vi "Insert Tag.vi"(0 "Image Data in":u8[](array[numeric]), 2 "Cluster":T1={"Tag"=30, "Type"=enum."RATIONAL", "Count"=2, "Val/Offs"=106, "Is Pointer?"=TRUE, "Byte stream index"=0}, 4 "Litt/BigEnd":bool) -> (5 "Image Data Out":u8[](array[numeric]))   [LabVIEW 2013, in "Tiff reader.lvlib"]
doc: "Sets a tag entry in the Image File Directory in a tiff file byte stream."
uses:
  Tiff reader.lvlib
  IFD Entry.ctl
  FieldTypes.ctl
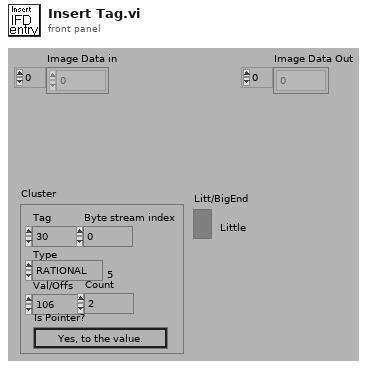
[diagram p1: front panel]
types:
  T1 = typedef "Tiff reader.lvlib/IFD Entry.ctl" = cluster{"Tag":u16, "Type":T2, "Count":u32, "Val/Offs":u32, "Is Pointer?":bool, "Byte stream index":i32}
  T2 = typedef "Tiff reader.lvlib/FieldTypes.ctl" = enum16{"NULL", "U8", "ASCII7", "U16", "U32", "RATIONAL", "SByte(I8)", "Undef(8Bit)", "I16", "I32", "SRat(4B:4B)", "SGL(4Byte)", "DBL(8Byte)"}
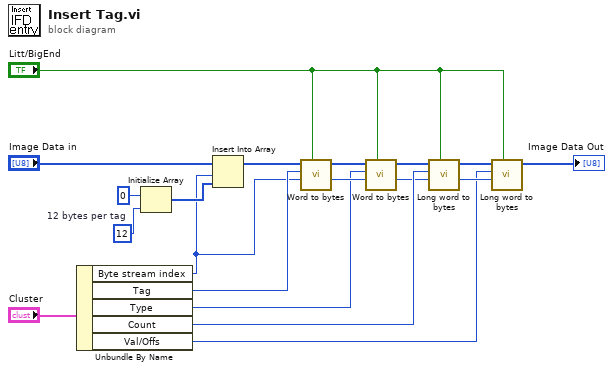
[diagram p0: block diagram]
diagram:
  w15 = 12  # 12 bytes per tag
  n1 = Unbundle By Name("Cluster") -> ("Byte stream index"=w1:i32, "Tag"=w18:u16, "Type"=w10:T2, "Count"=w9:u32, "Val/Offs"=w2:u32)
  n2 = Initialize Array(u8 0 ("Numeric"), w15) -> (w14:u8[])
  n3 = Insert Into Array "Insert Into Array"(array="Image Data in", index=w1, new element=w14) -> (w13:u8[])
  n4 = call "Word to bytes.vi"("Litt/BigEnd"="Litt/BigEnd", "Index"=w1, "Word"=w18, "Image Data in"=w13) -> ("Index+2"=w11:i32, "Image Data out"=w12:u8[])  [unwired: 4 out]
  n5 = call "Word to bytes.vi"("Litt/BigEnd"="Litt/BigEnd", "Index"=w11, "Word"=w10, "Image Data in"=w12) -> ("Index+2"=w8:i32, "Image Data out"=w6:u8[])  [unwired: 4 out]
  n6 = call "Long word to bytes.vi"("Litt/BigEnd"="Litt/BigEnd", "Index"=w8, "U32"=w9, "Image Data in"=w6) -> ("Index+4"=w7:i32, "Image Data out"=w4:u8[])  [unwired: 4 out]
  n7 = call "Long word to bytes.vi"("Litt/BigEnd"="Litt/BigEnd", "Index"=w7, "U32"=w2, "Image Data in"=w4) -> ("Image Data out"=→"Image Data Out":u8[])  [unwired: 5 out]
